vi "PathPlanner_ReadTrajectory_CSV_File_FGV_Example.vi"() -> ()   [LabVIEW 2019]
panel:
  out "error out":errorcluster
  # "Read Trajectory CSV File and Write to Functional Global Variable"
  # "See block diagram"
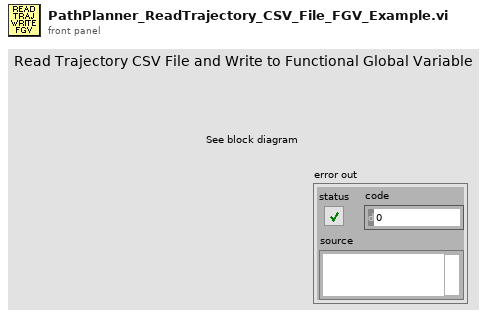
[diagram p1: front panel]
types:
  T1 = typedef "PathPlanner24.lvlib/PathPlannerTrajectory.ctl" = cluster{"States":T2[]}
  T2 = typedef "PathPlanner24.lvlib/PathPlannerTrajectoryState.ctl" = cluster{"TimeSeconds":dbl, "VelocityMPS":dbl, "AccerationMpsSq":dbl, "HeadingAngularVelRadPerSec":dbl, "PositionMeters":T3, "Heading":T4, "TargetHolonomicRotation":T4, "CurvatureRadPerMeter":dbl, "PathPlannerConstraints":T5, "DeltaPos":dbl}
  T3 = typedef "Trajectory_Library.lvlib/TRANSLATION2D.ctl" = cluster{"X":dbl, "Y":dbl}
  T4 = typedef "Trajectory_Library.lvlib/ROTATION2D.ctl" = cluster{"VALUE":dbl, "COS":dbl, "SIN":dbl}
  T5 = typedef "PathPlanner24.lvlib/PathPlannerPathConstraints.ctl" = cluster{"MaxVelocityMps;":dbl, "MaxAccelerationMpsSq;":dbl, "MaxAngularVelRadPsEc;":dbl, "MaxAngularAccRadPSecSq":dbl, "Exists":bool}
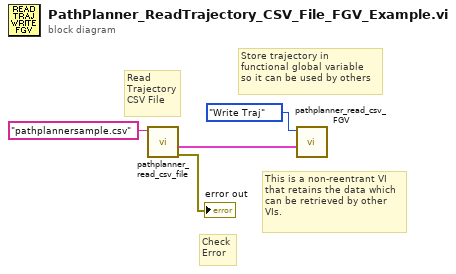
[diagram p0: block diagram]
diagram:
  # "Check\nError"
  # "This is a non-reentrant VI\nthat retains the data which\ncan be retrieved by other\nVIs."
  # "Read\nTrajectory\nCSV File"
  # "Store trajectory in\nfunctional global variable\nso it can be used by others"
  n1 = call "pathplanner_read_csv_file.vi"("CSV File Name"="pathplannersample.csv") -> ("error out"=→"error out":errorcluster, "Path Planner Trajectory"=w4:T1)  [unwired: 7 in, 2 out]
  n2 = call "pathplanner_read_csv_FGV.vi"("inTRAJECTORY"=w4, "Command"=enum16{"Sample", "Read Traj", "Write Traj"}."Write Traj") -> ()  [unwired: 8 in, 2 out]
